vi "Build Read.vi"(4 "Limit":i64, 6 "Where":string, 8 "error in (no error)":errorcluster, 9 "tableName":string, 10 "DynamicParameters in":refnum<class "DynamicParameters.lvclass">, 11 "DbConnection in":refnum<class "DbConnection.lvclass">) -> (0 "error out":errorcluster, 2 "Query":string, 3 "DbConnection out":refnum<class "DbConnection.lvclass">)   [LabVIEW 2020, in "ORM.lvlib" / "DbConnection.lvclass"]
uses:
  DbConnection.lvclass
  DynamicParameters/DynamicParameters.lvclass
  DbConnection.lvclass/DbConnection.ctl
  DynamicParameters/DynamicParameters.lvclass/DynamicParameters.ctl
  DynamicParameters/Read FieldNames.vi
  DynamicParameters/Read ParameterNames.vi
  Read ColumnNameEqualsValueFormat.vi
  <vilib>/regexp/Match Regular Expression.xnode
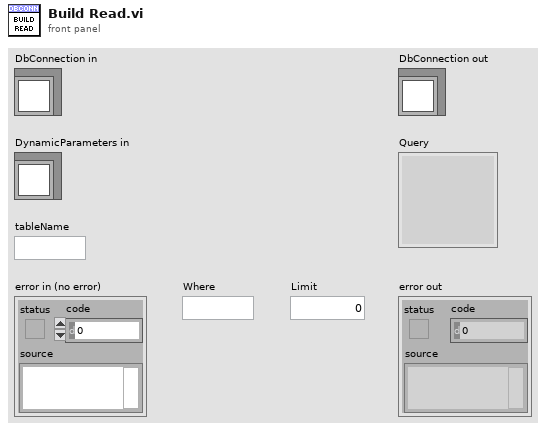
[diagram p1: front panel]
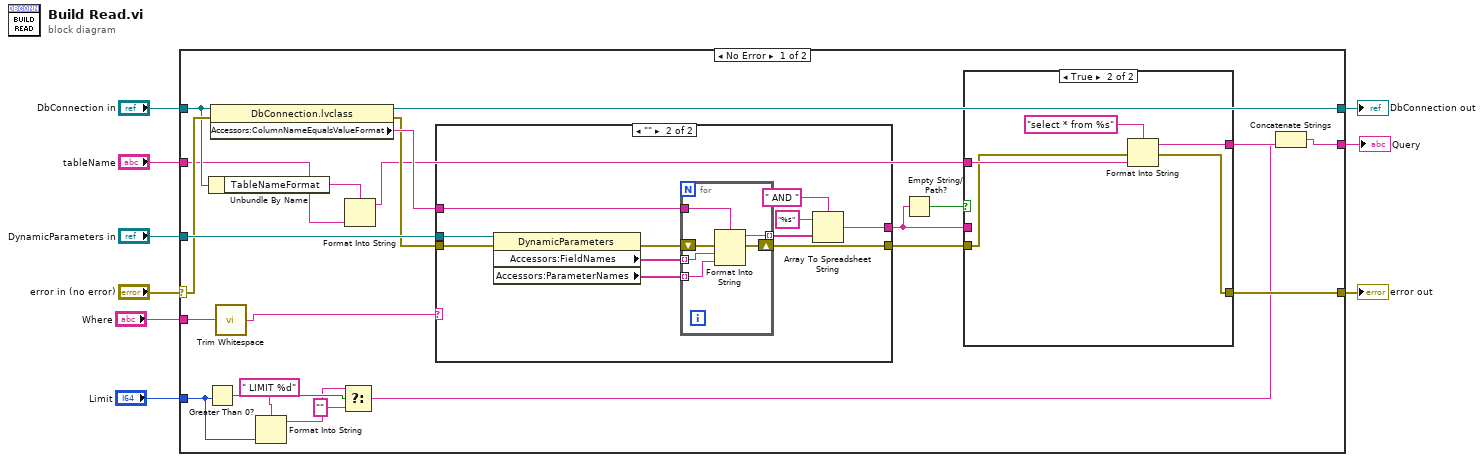
[diagram p0: block diagram]
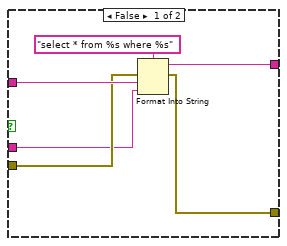
[diagram p2: hidden frame]
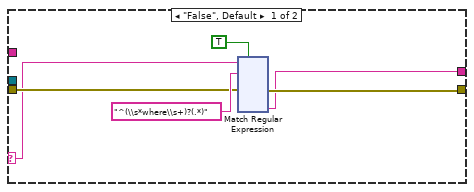
[diagram p3: hidden frame]
diagram:
  n1 = case shown="No Error" "error in (no error)" {
    selector: "error in (no error)" -> [w29 w185]
    tunnel: [w26 w185] -> w8
    tunnel: [w32 w184] -> w6
    tunnel: "DbConnection in" -> [w13 w184]
    tunnel: "DynamicParameters in" -> [w31 _]
    tunnel: "tableName" -> [w11 _]
    tunnel: [w14 _] -> w3
    tunnel: "Where" -> [w25 _]
    tunnel: "Limit" -> [w21 _]
    frame No Error {
      n2 = Greater Than 0?(x=w21) -> (x > 0?=w19:bool)
      n3 = Unbundle By Name(w13) -> ("TableNameFormat"=w12:string)
      n4 = property class="DbConnection.lvclass"(reference=w13, error in=w29) -> (reference out=w32:refnum<class "DbConnection.lvclass">, error out=w28:errorcluster, "Accessors:ColumnNameEqualsValueFormat"=w30:string)
      n5 = call <vilib>:"Trim Whitespace.vi"("string"=w25) -> ("trimmed string"=w24:string)  [unwired: 1 in]
      n6 = Format Into String(format string=" LIMIT %d", w21) -> (resulting string=w18:string)  [unwired: 2 in, 1 out]
      n7 = Select(t=w18, s=w19, f="") -> (s? t:f=w15:string)
      n8 = Format Into String(format string=w12, w11) -> (resulting string=w10:string)  [unwired: 2 in, 1 out]
      n9 = case shown="\"\"" w24 {
        selector: w24 -> [w45 _]
        tunnel: w31 -> [_ w177]
        tunnel: w30 -> [_ w174]
        tunnel: [w44 w173] -> w23
        tunnel: w28 -> [w47 w169]
        tunnel: [w46 w167] -> w27
        frame "False", Default {
          n10 = xnode "Match Regular Expression"("input string"=w45, "regular expression"="^(\\s*where\\s+)?(.*)", "error in"=w47, "ignore case? (F)"=TRUE) -> ("error out"=w46:errorcluster, "submatch 2"=w44:string)  [unwired: 2 in, 5 out]
        }
        frame "" {
          n11 = property class="DynamicParameters"(reference=w177, error in=w169) -> (error out=w168:errorcluster, "Accessors:FieldNames"=w176:string[], "Accessors:ParameterNames"=w175:string[])  [unwired: 1 out]
          n12 = for {
            tunnel: w176 -> [w182] mode=indexing
            tunnel: w175 -> [w181] mode=indexing
            tunnel: w174 -> [w183]
            tunnel: [w180] -> w171 mode=indexing
            shift-right: [w178] -> w167
            shift-left: w168 -> [w179]
            n13 = Format Into String(format string=w183, error in=w179, w182, w181) -> (resulting string=w180:string, error out=w178:errorcluster)  [unwired: 1 in]
          }
          n14 = Array To Spreadsheet String(delimiter (Tab)=" AND ", array=w171, 3:"%s" ("format string")) -> (spreadsheet string=w173:string)
        }
      }
      n15 = Empty String/Path?(string/path=w23) -> (empty?=w22:bool)
      n16 = case shown="True" w22 {
        tunnel: w10 -> [w37 w42]
        tunnel: [w36 w40] -> w16
        tunnel: w27 -> [w35 w39]
        tunnel: [w34 w41] -> w26
        tunnel: w23 -> [w33 _]
        frame False {
          n17 = Format Into String(format string="select * from %s where %s", error in=w35, w37, w33) -> (resulting string=w36:string, error out=w34:errorcluster)  [unwired: 1 in]
        }
        frame True {
          n18 = Format Into String(format string="select * from %s", error in=w39, w42) -> (resulting string=w40:string, error out=w41:errorcluster)  [unwired: 1 in]
        }
      }
      n19 = Concatenate Strings(w16, w15) -> (w14:string)
    }
    frame Error {
    }
  }
  "error out" <- w8
  "DbConnection out" <- w6
  "Query" <- w3
